vi "Open Connection to Actuator.vi"(8 "error in (no error)":errorcluster, 11 "VISA resource name":refnum<visa-resource-name>) -> (0 "error out":errorcluster, 3 "VISA resource name out":refnum<visa-resource-name>)   [LabVIEW 2018]
doc: "Opens a connection to the VICI universal electric actuator.\n\n\n(Nimble Focus Consulting 2019)"
uses:
  <vilib>/Instr/_visa.llb/VISA Configure Serial Port (Instr).vi
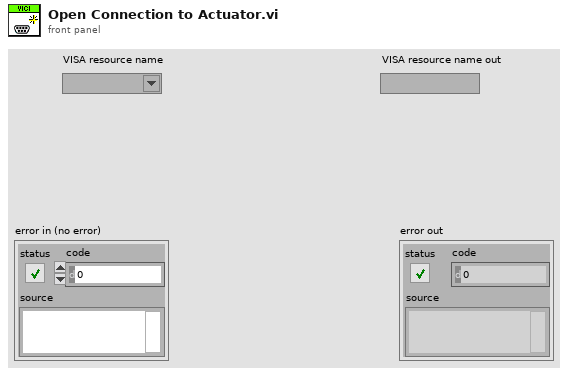
[diagram p1: front panel]
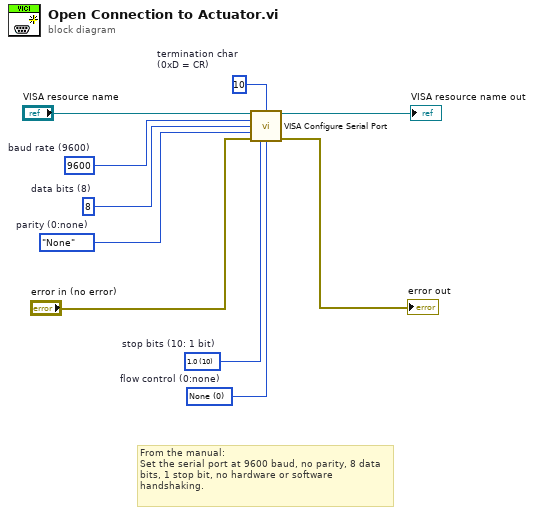
[diagram p0: block diagram]
diagram:
  w1 = u8 10  # termination char (0xD = CR)
  w4 = u16 0 items=["None", "XON/XOFF", "RTS/CTS", "XON/XOFF & RTS/CTS", "DTR/DSR", "XON/XOFF & DTR/DSR"]  # flow control (0:none)
  w5 = u16 10 items=["1.0"=10, "1.5"=15, "2.0"=20]  # stop bits (10: 1 bit)
  w6 = enum16{"None", "Odd", "Even", "Mark", "Space"}."None"  # parity (0:none)
  w7 = u16 8  # data bits (8)
  w8 = u32 9600  # baud rate (9600)
  # "From the manual:\nSet the serial port at 9600 baud, no parity, 8 data\nbits, 1 stop bit, no hardware or software\nhandshaking."
  n1 = call-poly "VISA Configure Serial Port"("VISA resource name"="VISA resource name", "termination char\n(0xA = '\\n' = LF)"=w1, "baud rate (9600)"=w8, "data bits (8)"=w7, "parity (0:none)"=w6, "error in (no error)"="error in (no error)", "stop bits (10: 1 bit)"=w5, "flow control (0:none)"=w4) -> ("VISA resource name out"=→"VISA resource name out":refnum<visa-resource-name>, "error out"=→"error out":errorcluster)  [unwired: 6 in]
